vi "Angle to Encoder Ticks.vi"(2 "Angle(degrees)":dbl, 3 "Dart Length(in)":dbl) -> (0 "Dart Length(in)":dbl, 1 "Angle(degrees)":dbl)   [LabVIEW 2015]
doc: "Changes angle to dart length or dart length to angle."
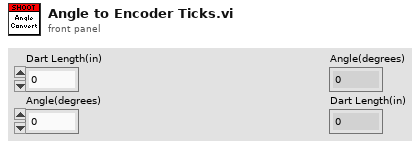
[diagram p1: front panel]
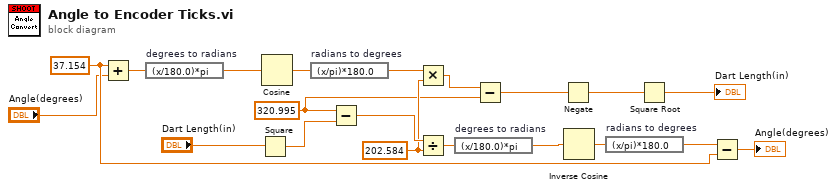
[diagram p0: block diagram]
diagram:
  w11 = 320.995 ("y")
  w17 = 37.154 ("y")
  w16 = 202.584 ("y")
  n1 = Add(x=w17, y="Angle(degrees)") -> (x+y=w5:dbl)
  n2 = expression code="(x/180.0)*pi" "degrees to radians"(w5) -> (w4:dbl)
  n3 = Square(x="Dart Length(in)") -> (x^2=w18:dbl)
  n4 = Cosine(x=w4) -> (cos(x)=w2:dbl)
  n5 = expression code="(x/pi)*180.0" "radians to degrees"(w2) -> (w1:dbl)
  n6 = Subtract(x=w11, y=w18) -> (x-y=w19:dbl)
  n7 = Multiply(x=w1, y=w16) -> (x*y=w15:dbl)
  n8 = Divide(x=w19, y=w16) -> (x/y=w7:dbl)
  n9 = expression code="(x/180.0)*pi" "degrees to radians"(w7) -> (w6:dbl)
  n10 = Subtract(x=w15, y=w11) -> (x-y=w13:dbl)
  n11 = Negate(x=w13) -> (-x=w14:dbl)
  n12 = Inverse Cosine(1:w6) -> (0:w10:dbl)
  n13 = expression code="(x/pi)*180.0" "radians to degrees"(w10) -> (w9:dbl)
  n14 = Square Root(x=w14) -> (sqrt(x)=→"Dart Length(in)":dbl)
  n15 = Subtract(x=w9, y=w17) -> (x-y=→"Angle(degrees)":dbl)
